vi "Set Joint Angles.vi"(8 "error in (no error)":errorcluster, 10 "motor_angles":dbl[](array[numeric]), 11 "Finger in":refnum<class "Finger.lvclass">) -> (0 "error out":errorcluster, 3 "Finger out":refnum<class "Finger.lvclass">)   [LabVIEW 2011, in "Finger.lvclass"]
uses:
  Finger.lvclass
  Finger.lvclass/Finger.ctl
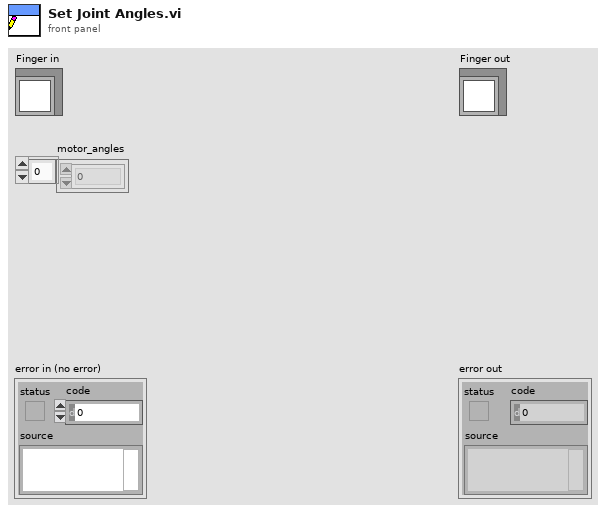
[diagram p1: front panel]
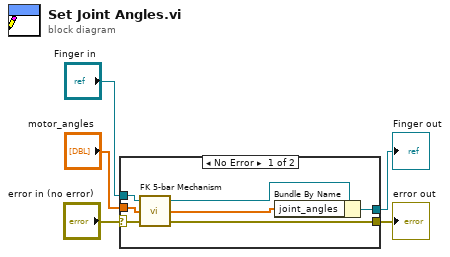
[diagram p0: block diagram]
diagram:
  n1 = case shown="No Error" "error in (no error)" {
    selector: "error in (no error)" -> [w7 w13]
    tunnel: [w6 w13] -> w4
    tunnel: [w12 w14] -> w2
    tunnel: "Finger in" -> [w9 w14]
    tunnel: "motor_angles" -> [w11 _]
    frame No Error {
      n2 = call "FK 5-bar Mechanism.vi"("error in (no error)"=w7, "motors angles"=w11, "Finger in"=w9) -> ("error out"=w6:errorcluster, "joint angles"=w10:dbl[], "Finger out"=w8:refnum<class "Finger.lvclass">)
      n3 = Bundle By Name(cluster=w8, "joint_angles"=w10) -> (w12:refnum<class "Finger.lvclass">)
    }
    frame Error {
    }
  }
  "error out" <- w4
  "Finger out" <- w2
